vi "Write Displays.vi"(5 "Displays":refnum<class "Digital.lvclass">[](array[class]), 9 "NumericWithScale in":refnum<class "NumericWithScale.lvclass">) -> (3 "NumericWithScale out":refnum<class "NumericWithScale.lvclass">)   [LabVIEW 2014, in "Raspberry Pi Compatible Compiler for LabVIEW.lvlib" / "NumericWithScale.lvclass"]
uses:
  NumericWithScale.lvclass
  Digital/Digital.lvclass
  NumericWithScale.lvclass/NumericWithScale.ctl
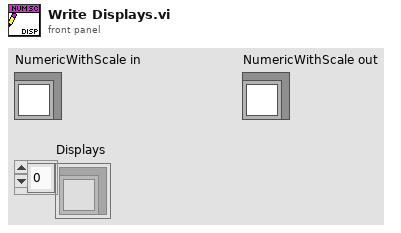
[diagram p1: front panel]
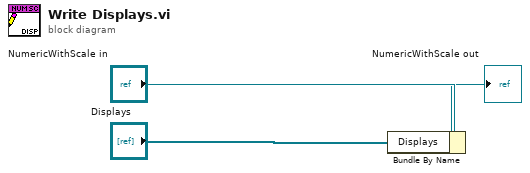
[diagram p0: block diagram]
diagram:
  n1 = Bundle By Name(cluster="NumericWithScale in", "Displays"="Displays") -> (→"NumericWithScale out":refnum<class "NumericWithScale.lvclass">)
